vi "Update Logger List.vi"(8 "error in (no error)":errorcluster, 11 "MulticolumnListbox in":refnum<vi>) -> (0 "error out":errorcluster)   [LabVIEW 2018]
uses:
  api/GLog.lvlib
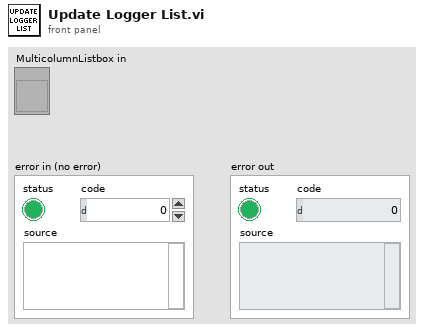
[diagram p1: front panel]
types:
  T1 = typedef "GLog.lvlib/Log Levels.ctl" = enum16{"Trace", "Debug", "Info", "Warning", "Error", "Critical"}
  T2 = cluster{"Name":string, "Minimum Log Level":T1, "Enabled?":bool}[]
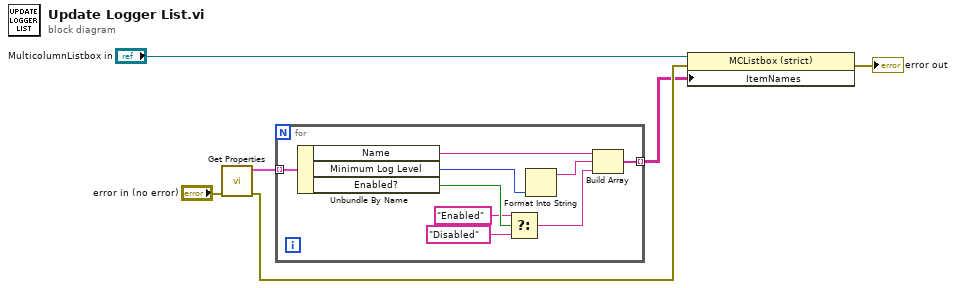
[diagram p0: block diagram]
diagram:
  n1 = call "Get Properties.vi"("error in"="error in (no error)") -> ("error out"=w5:errorcluster, "logger info"=w3:T2)  [unwired: 9 in]
  n2 = for {
    tunnel: w3 -> [w15] mode=indexing
    tunnel: [w7] -> w4 mode=indexing
    n3 = Unbundle By Name(w15) -> ("Name"=w10:string, "Minimum Log Level"=w11:T1, "Enabled?"=w14:bool)
    n4 = Select(t="Enabled", s=w14, f="Disabled") -> (s? t:f=w8:string)
    n5 = Format Into String(w11) -> (resulting string=w9:string)  [unwired: 3 in, 1 out]
    n6 = Build Array(w10, w9, w8) -> (w7:string[])
  }
  n7 = property class="MCListbox (strict)"(reference="MulticolumnListbox in", error in=w5, "ItemNames"=w4) -> (error out=→"error out":errorcluster)  [unwired: 1 out]
